vi "LCD Scroll Display.vi"(0 "Arduino Resource":T1, 7 "Direction":T3, 11 "error in":errorcluster) -> (4 "Arduino Resource":T1, 15 "error out":errorcluster)   [LabVIEW 2011, in "LabVIEW Interface for ChipKit.lvlib"]
doc: "Scrolls the display one space in the direction specified."
uses:
  <vilib>/LabVIEW Interface for ChipKit/LabVIEW Interface for ChipKit.lvlib
  <vilib>/LabVIEW Interface for ChipKit/Private/Type Defs/Chipkit Resource.ctl
  <vilib>/LabVIEW Interface for ChipKit/Private/Type Defs/Board Type.ctl
  <vilib>/LabVIEW Interface for ChipKit/Private/Type Defs/Direction.ctl
  <vilib>/LabVIEW Interface for ChipKit/Private/Type Defs/Command.ctl
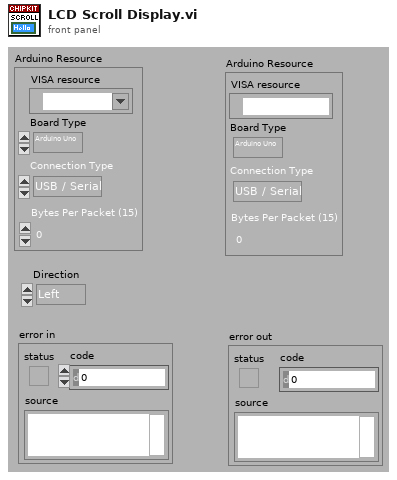
[diagram p1: front panel]
types:
  T1 = typedef "LabVIEW Interface for ChipKit.lvlib/Chipkit Resource.ctl" = cluster{"VISA resource":refnum<visa-resource-name>, "Board Type":T2, "Connection Type":enum8{"USB / Serial"}, "Bytes Per Packet (15)":u8}
  T2 = typedef "LabVIEW Interface for ChipKit.lvlib/Board Type.ctl" = enum16{"Arduino Uno", "Dimuelanove w/Atmega 328", "Mega 2560", "Chipkit Uno32", "Chipkit Max32"}
  T3 = typedef "LabVIEW Interface for ChipKit.lvlib/Direction.ctl" = enum8{"Left ", "Right"}
  T4 = typedef "LabVIEW Interface for ChipKit.lvlib/Command.ctl" = enum8{"setArduinoMode", "flushSerial", "setPinMode", "digitalWritePin", "digitalWritePort", "tone", "digitalReadPin", "digitalReadPort", "analogReadPin", "analogReadPort", "pwmWritePin", "pwmWritePort", "sevenSegment_Configure", "sevenSegment_Write", "I2C Init", "I2C Write", "I2C Read", "SPI Init", "SPI Set Bit Order", "SPI Set Clock Divider", "SPI Set Data Mode", "SPI Send / Receive", "SPI Close", "Servo Set Num Servos", "Servo Config Servo", "Servo Write Angle", "Servo Read Angle", "Servo Write Pulse Width", "Servo Read Pulse Width", "Servo Detach", "LCD Init", "LCD Set Size", "LCD Set Cursor Mode", "LCD Clear", "LCD Set Cursor Position", "LCD Print", "LCD Display Power", "LCD Scroll Display", "LCD Autoscroll", "LCD Print Direction", "LCD Create Custom Char", "LCD Print Custom Char", "contAcqOn", "contAcqOff", "getFirmwareVersion", "FiniteSampleStart"}
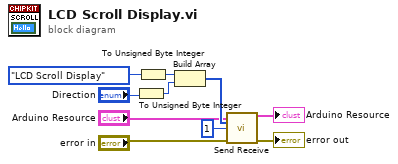
[diagram p0: block diagram]
diagram:
  n1 = To Unsigned Byte Integer(number="Direction") -> (unsigned 8bit integer=w1:u8)
  n2 = To Unsigned Byte Integer(number=Command."LCD Scroll Display" ("Command")) -> (unsigned 8bit integer=w5:u8)
  n3 = Build Array(w5, w1) -> (w7:u8[])
  n4 = call <vilib>:"Send Receive.vi"("Arduino Resource"="Arduino Resource", "Data"=w7, "Bytes To Read (0)"=u8 1, "error in"="error in") -> ("Arduino Resource"=→"Arduino Resource":T1, "error out"=→"error out":errorcluster)  [unwired: 9 in, 1 out]
